vi "Default Case.vi"(7 "Default Case":bool, 10 "Boolean in":bool) -> (2 "Boolean out":bool)   [LabVIEW 2016]
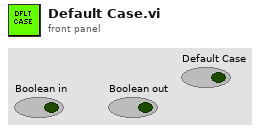
[diagram p1: front panel]
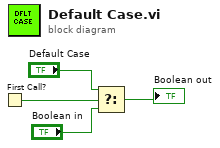
[diagram p0: block diagram]
diagram:
  n1 = First Call?() -> (First Call?: T/F=w3:bool)
  n2 = Select(t="Default Case", s=w3, f="Boolean in") -> (s? t:f=→"Boolean out":bool)
